vi "Parameter - Supra.vi"() -> ()   [LabVIEW 2016, in "NI-PCG Vehicle Model.lvlib"]
uses:
  NI-PCG Vehicle Model.lvlib
  Types/Engine Parameters.ctl
  Types/Transmission Parameters.ctl
  Types/Vehicle Parameters.ctl
panel:
  in  "Supra Parameters":T4={"Engine Parameters"={"Ambient Parameters"={"Temperature (K)"=288.0, "Pressure (Pa)"=101325.01}, "Air Parameters"={"R (Ideal Gas Constant)"=287.05, "Molecular Weight"=28.964, "Cp (Specific Heat Constant)"=1005.0, "Density (kg/m^3)"=1.229, "Stoichiometric A/F Ratio"=14.7}, "Engine Geometry Parameters"={"Cylinder Volume (l)"=2.997, "J (Rotational Moment of Inertia)"=0.14, "Minimuim Engine Speed"=73.304, "Maximum Engine Speed"=785.398, "Intake Manifold Volume (l)"=6.0}, "Volumetric Efficiency Map"={"MAP"=[0.0, 0.2, 0.3, 0.35, 0.4, 0.45, 0.55, 0.65, 0.75, 0.85, 0.95, 1.0, 1.16, 1.32, 1.48, 1.64, 1.8], "RPM"=[800.0, 1000.0, 1300.0, 1600.0, 1900.0, 2300.0, 2700.0, 3200.0, 3600.0, 4000.0, 4400.0, 4800.0, 5200.0, 5600.0, 6550.0, 7500.0], "Table"=[[0.01, 0.01, 0.01, 0.01, 0.01, 0.01, 0.01, 0.01, 0.01, 0.01, 0.01, 0.01, 0.01, 0.01, 0.01, 0.01], [0.506, 0.508, 0.512, 0.52, 0.534, 0.559, 0.591, 0.635, 0.666, 0.69, 0.703, 0.703, 0.689, 0.672, 0.655, 0.639], [0.511, 0.519, 0.541, 0.576, 0.621, 0.686, 0.745, 0.801, 0.829, 0.84, 0.836, 0.818, 0.797, 0.778, 0.758, 0.739], [0.516, 0.531, 0.568, 0.62, 0.678, 0.751, 0.811, 0.761, 0.882, 0.888, 0.879, 0.857, 0.835, 0.814, 0.794, 0.774], [0.528, 0.549, 0.604, 0.669, 0.734, 0.808, 0.864, 0.908, 0.925, 0.927, 0.914, 0.891, 0.869, 0.847, 0.826, 0.805], [0.538, 0.573, 0.643, 0.727, 0.784, 0.856, 0.908, 0.948, 0.962, 0.961, 0.946, 0.922, 0.899, 0.877, 0.855, 0.833], [0.582, 0.64, 0.729, 0.807, 0.87, 0.936, 0.928, 1.017, 1.027, 1.023, 1.005, 0.98, 0.955, 0.931, 0.908, 0.885], [0.645, 0.715, 0.807, 0.88, 0.94, 1.002, 1.046, 1.078, 1.087, 1.081, 1.061, 1.034, 1.008, 0.983, 0.958, 0.934], [0.709, 0.781, 0.87, 0.94, 0.998, 1.052, 1.103, 1.135, 1.144, 1.138, 1.115, 1.087, 1.06, 1.033, 1.008, 0.982], [0.768, 0.838, 0.924, 0.994, 1.052, 1.113, 1.158, 1.191, 1.2, 1.192, 1.169, 1.14, 1.111, 1.083, 1.056, 1.03], [0.789, 0.853, 0.933, 1.001, 1.057, 1.118, 1.162, 1.195, 1.203, 1.195, 1.172, 1.142, 1.114, 1.086, 1.059, 1.032], [0.829, 0.895, 0.978, 1.047, 1.106, 1.169, 1.215, 1.249, 1.258, 1.25, 1.225, 1.194, 1.165, 1.135, 1.107, 1.079], [0.944, 1.013, 1.103, 1.179, 1.244, 1.314, 1.366, 1.403, 1.413, 1.404, 1.376, 1.342, 1.308, 1.275, 1.243, 1.212], [1.034, 1.106, 1.202, 1.284, 1.354, 1.43, 1.485, 1.526, 1.537, 1.528, 1.497, 1.459, 1.423, 1.387, 1.352, 1.319], [1.101, 1.176, 1.275, 1.362, 1.436, 1.516, 1.575, 1.619, 1.629, 1.619, 1.587, 1.547, 1.508, 1.471, 1.434, 1.398], [1.145, 1.222, 1.324, 1.414, 1.491, 1.574, 1.635, 1.68, 1.691, 1.68, 1.647, 1.605, 1.565, 1.526, 1.488, 1.451], [1.167, 1.244, 1.348, 1.439, 1.518, 1.602, 1.664, 1.71, 1.721, 1.71, 1.676, 1.634, 1.593, 1.553, 1.515, 1.477]]}, "Fuel LHV (J/kg)"=42700000.0, "Combustion Efficiency Map"={"Spark Timing (deg BTDC))"=[0.0, 25.0, 50.0], "Engine Speed (RPM)"=[200.0, 6200.0], "Combustion Efficiency"=[[0.75, 0.75], [1.0, 1.0], [0.75, 0.75]]}, "Thermodynamic Efficiency"=0.4}, "Transmission Parameters"={"Final Drive Ratio"=3.266, "Transmission Gear Ratios"={"Gears"=[1.0, 2.0, 3.0, 4.0, 5.0, 6.0], "Gear Ratios"=[3.827, 2.36, 1.685, 1.312, 1.0, 0.793]}, "Torque Converter Map"={"Speed Ratio"=[0.0, 0.1, 0.2, 0.3, 0.4, 0.5, 0.6, 0.7, 0.8, 0.81, 0.82, 0.83, 0.84, 0.85, 0.86, 0.87, 0.88, 0.89, 0.9, 0.92, 0.94, 0.97], "K Factor"=[18.9894, 18.9341, 18.7683, 18.7407, 19.0033, 19.3902, 20.0674, 21.1178, 22.5137, 22.6933, 22.9559, 23.2047, 23.4949, 23.8681, 24.2274, 24.8079, 25.3607, 26.2314, 27.3094, 29.8247, 33.7774, 100.0], "Torque Ratio"=[2.232, 2.075, 1.975, 1.846, 1.72, 1.564, 1.409, 1.254, 1.096, 1.08, 1.061, 1.043, 1.028, 1.012, 1.002, 1.002, 1.001, 0.998, 0.997, 0.996, 0.995, 0.994]}, "Upshift Throttle"=[0.0, 25.0, 35.0, 50.0, 90.0, 100.0], "Downshift Throttle"=[0.0, 5.0, 40.0, 50.0, 90.0, 100.0], "Upshift Table"=[[10.0, 20.0, 30.0, 40.0, 50.0, 1000000.0], [10.0, 20.0, 30.0, 40.0, 50.0, 1000000.0], [15.0, 23.0, 30.0, 40.0, 50.0, 1000000.0], [23.0, 32.0, 41.0, 51.0, 60.0, 1000000.0], [40.0, 1000000.0, 1000000.0, 1000000.0, 1000000.0, 1000000.0], [40.0, 1000000.0, 1000000.0, 1000000.0, 1000000.0, 1000000.0]], "Downshift Table"=[[0.0, 5.0, 13.0, 20.0, 28.0, 35.0], [0.0, 5.0, 13.0, 20.0, 28.0, 35.0], [0.0, 5.0, 25.0, 25.0, 33.0, 40.0], [0.0, 5.0, 28.0, 30.0, 40.0, 50.0], [0.0, 30.0, 40.0, 50.0, 65.0, 80.0], [0.0, 30.0, 40.0, 50.0, 65.0, 80.0]], "Wait Time"=2}, "Vehicle Parameters"={"Vehicle Mass (kg)"=1590.0, "Vehicle Cd"=0.33, "Vehicle Frontal Area (m^2)"=2.308, "Wheel Radius (m)"=0.3178, "Wheel Rolling Resistance"=0.012}} {"Engine Parameters"."Engine Geometry Parameters"."Intake Manifold Volume (l)" format="%#_6p"}
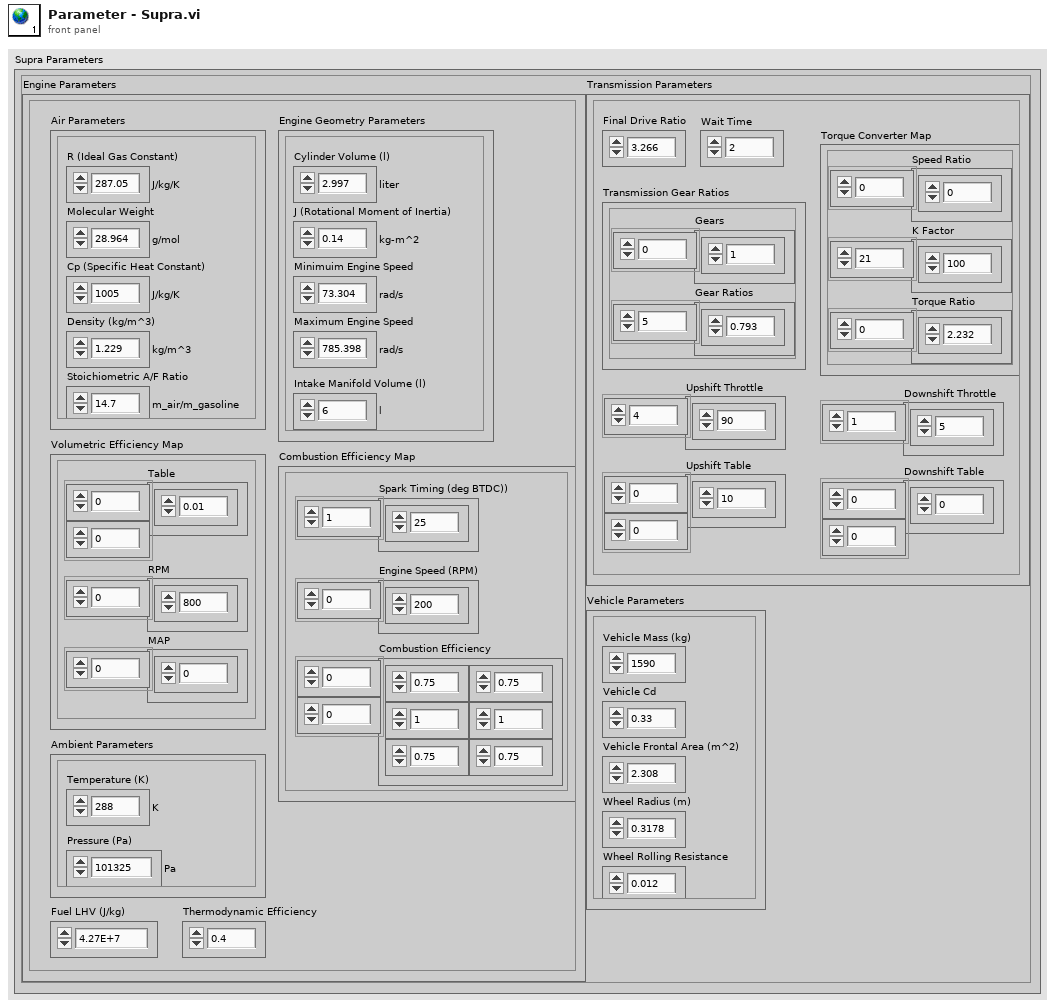
[diagram p1: front panel]
types:
  T1 = typedef "NI-PCG Vehicle Model.lvlib/Engine Parameters.ctl" = cluster{"Ambient Parameters":cluster{"Temperature (K)":sgl, "Pressure (Pa)":sgl}, "Air Parameters":cluster{"R (Ideal Gas Constant)":sgl, "Molecular Weight":sgl, "Cp (Specific Heat Constant)":sgl, "Density (kg/m^3)":sgl, "Stoichiometric A/F Ratio":sgl}, "Engine Geometry Parameters":cluster{"Cylinder Volume (l)":sgl, "J (Rotational Moment of Inertia)":sgl, "Minimuim Engine Speed":sgl, "Maximum Engine Speed":sgl, "Intake Manifold Volume (l)":sgl}, "Volumetric Efficiency Map":cluster{"MAP":sgl[], "RPM":sgl[], "Table":sgl[][]}, "Fuel LHV (J/kg)":sgl, "Combustion Efficiency Map":cluster{"Spark Timing (deg BTDC))":sgl[], "Engine Speed (RPM)":sgl[], "Combustion Efficiency":sgl[][]}, "Thermodynamic Efficiency":sgl}
  T2 = typedef "NI-PCG Vehicle Model.lvlib/Transmission Parameters.ctl" = cluster{"Final Drive Ratio":sgl, "Transmission Gear Ratios":cluster{"Gears":sgl[], "Gear Ratios":sgl[]}, "Torque Converter Map":cluster{"Speed Ratio":sgl[], "K Factor":sgl[], "Torque Ratio":sgl[]}, "Upshift Throttle":sgl[], "Downshift Throttle":sgl[], "Upshift Table":sgl[][], "Downshift Table":sgl[][], "Wait Time":u8}
  T3 = typedef "NI-PCG Vehicle Model.lvlib/Vehicle Parameters.ctl" = cluster{"Vehicle Mass (kg)":sgl, "Vehicle Cd":sgl, "Vehicle Frontal Area (m^2)":sgl, "Wheel Radius (m)":sgl, "Wheel Rolling Resistance":sgl}
  T4 = cluster{"Engine Parameters":T1, "Transmission Parameters":T2, "Vehicle Parameters":T3}
diagram:
